vi "Handle Value Change.vi"(7 "PrevLog":string, 10 "NewVal":variant, 11 "Ctl Refnum":refnum<vi>) -> (5 "Log":string)   [LabVIEW 2020, in "NoCodeEngine.lvlib"]
uses:
  NoCodeEngine.lvlib
  <vilib>/Utility/Data Type/NI_Data Type.lvlib
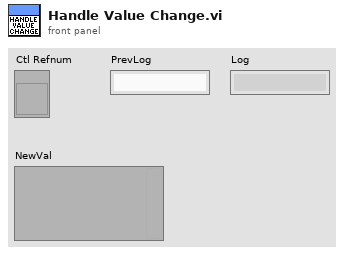
[diagram p1: front panel]
types:
  T1 = typedef "NI_Data Type.lvlib/Data Type.ctl" = enum8{"Invalid Type", "Void", "I8", "I16", "I32", "I64", "U8", "U16", "U32", "U64", "Single Float", "Double Float", "Extended Float", "Single Complex", "Double Complex", "Extended Complex", "Enum U8", "Enum U16", "Enum U32", "Enum U64", "Single Float With Unit", "Double Float With Unit", "Extended Float With Unit", "Single Complex with Unit", "Double Complex with Unit", "Extended Complex with Unit", "Boolean", "String", "Path", "Picture", "Tag", "Array", "Cluster", "Variant", "LV Variant", "Waveform", "Timestamp", "Digital Waveform", "Digital Data", "ExpressData", "Refnum", "External Data", "VI", "Poly VI", "LabVIEW Class Instance", "Fixed Point", "Set Collection", "Map Collection"}
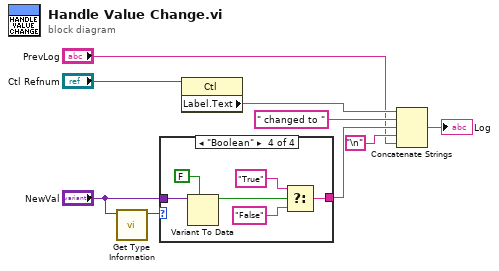
[diagram p0: block diagram]
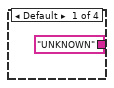
[diagram p2: hidden frame]
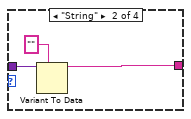
[diagram p3: hidden frame]
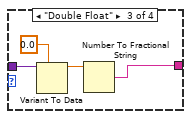
[diagram p4: hidden frame]
diagram:
  n1 = call <vilib>:"Get Type Information.vi"("variant"="NewVal") -> ("type"=w9:T1)  [unwired: 6 in, 4 out]
  n2 = case shown="\"Boolean\"" w9 {
    tunnel: "NewVal" -> [_ w13 w17 w23]
    tunnel: ["UNKNOWN" w11 w14 w18] -> w6
    frame Default {
    }
    frame "String" {
      n3 = Variant To Data(type="", Variant=w13) -> (data=w11:string)  [unwired: 1 in, 1 out]
    }
    frame "Double Float" {
      n4 = Variant To Data(type=0.0, Variant=w17) -> (data=w15:dbl)  [unwired: 1 in, 1 out]
      n5 = Number To Fractional String(number=w15) -> (F-format string=w14:string)  [unwired: 3 in]
    }
    frame "Boolean" {
      n6 = Variant To Data(type=FALSE, Variant=w23) -> (data=w21:bool)  [unwired: 1 in, 1 out]
      n7 = Select(t="True", s=w21, f="False") -> (s? t:f=w18:string)
    }
  }
  n8 = property class="Ctl"(reference="Ctl Refnum") -> ("Label.Text"=w8:string)  [unwired: 1 in, 2 out]
  n9 = Concatenate Strings(w8, " changed to " ("string"), w6, "\n", "PrevLog") -> (→"Log":string)
